vi "Server_Detect.vi"(8 "error in":errorcluster, 11 "Main Update Data":T1) -> (0 "error out":errorcluster)   [LabVIEW 2018, in "Cloud Server.lvlib"]
uses:
  Cloud Server.lvlib
  Data Def/Server_Main Update Data.ctl
  Data Def/Server_Connection Manager Method.ctl
  Com VIs/Data Def/Update Result.ctl
  Data Def/Server_Main Loop Queue Data.ctl
  Data Def/Server_Main Loop State.ctl
  Com VIs/Data Def/Data File Format.ctl
  <vilib>/gmath/NI_Gmath.lvlib
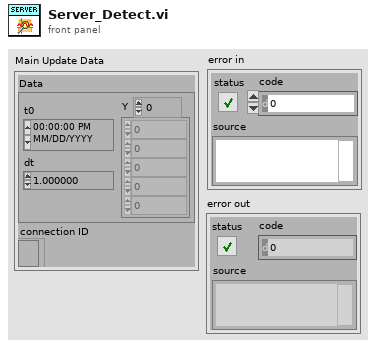
[diagram p1: front panel]
types:
  T1 = typedef "Cloud Server.lvlib/Server_Main Update Data.ctl" = cluster{"Data":waveform(dbl), "connection ID":refnum<k5>}
  T2 = typedef "Cloud Server.lvlib/Server_Connection Manager Method.ctl" = enum16{"Initialize", "Add", "Get", "Set Properties", "Get Properties", "Close", "Release"}
  T3 = typedef "Cloud Server.lvlib/Server_Connection Properties.ctl" = cluster{"User Data":T4, "Data":waveform(dbl)}
  T4 = typedef "User Data.ctl" = cluster{"Name":string, "Email":string, "Phone Number":string, "User Picture":u32[][], "Last Login Time":timestamp}
  T5 = typedef "Update Result.ctl" = enum16{"Normal", "Abnormal", "Can't find training data"}
  T6 = typedef "Data File Format.ctl" = cluster{"Data":waveform(dbl), "Abnormal?":bool, "Measure Time":timestamp, "User Name":string}
  T7 = typedef "Cloud Server.lvlib/Server_Main Loop Queue Data.ctl" = cluster{"Main Loop State":T8, "Data":variant}
  T8 = typedef "Cloud Server.lvlib/Server_Main Loop State.ctl" = enum16{"Detect", "Save", "Training", "Refresh User Name", "Stop"}
  T9 = typedef "Cloud Server.lvlib/Server_Training Data.ctl" = cluster{"Data":waveform(dbl), "Abnormal?":bool}
  T10 = typedef "Cloud Server.lvlib/Server_Main Data.ctl" = cluster{"Main VI Ref.":refnum<vi>, "Listener ID":refnum<k5>, "Meta data":T11[], "Main Queue":T13, "User Picture":T14}
  T11 = typedef "stm_MetaElement.ctl" = cluster{"Name":T12}
  T12 = typedef "stm_MetaDataElement.ctl" = string
  T13 = typedef "Cloud Server.lvlib/Server_Main Queue.ctl" = cluster{"Server Write Queue":refnum<queue>, "Main Loop Queue":refnum<queue>}
  T14 = typedef "IMAQ Image.ctl" = refnum<image>
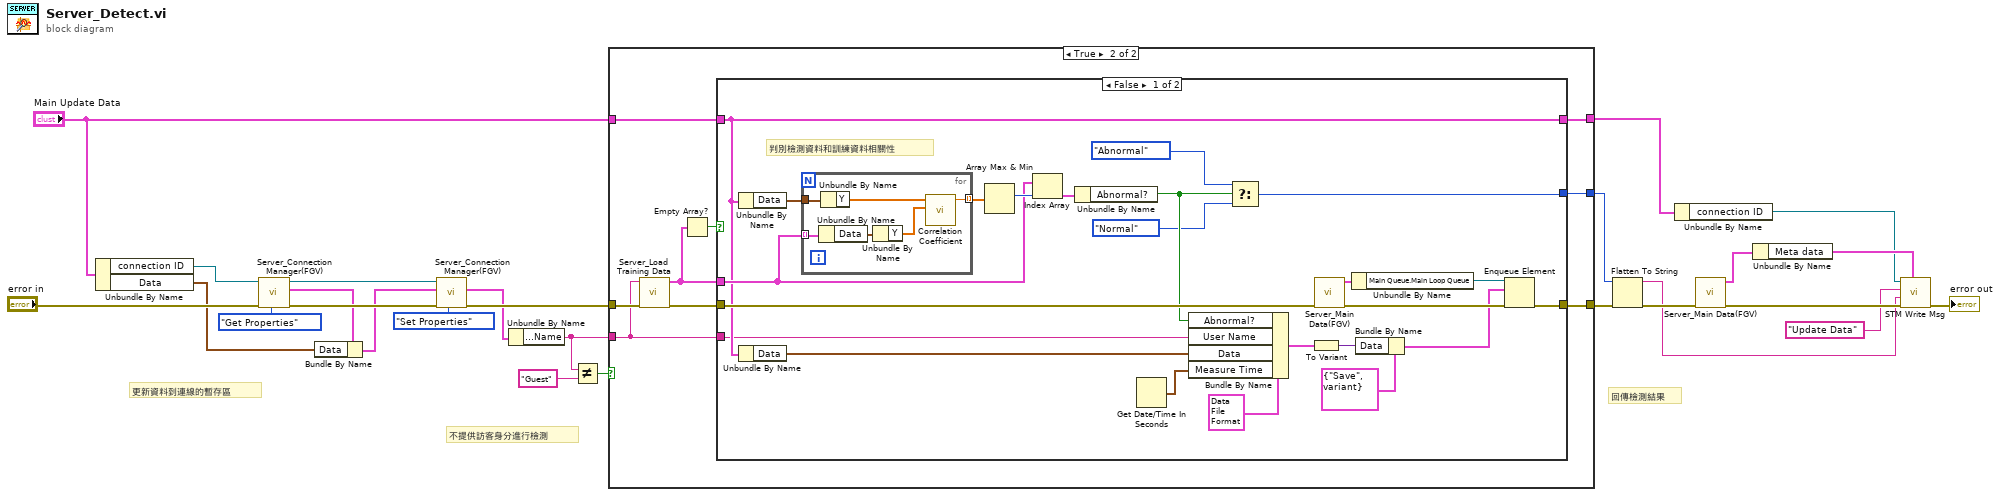
[diagram p0: block diagram]
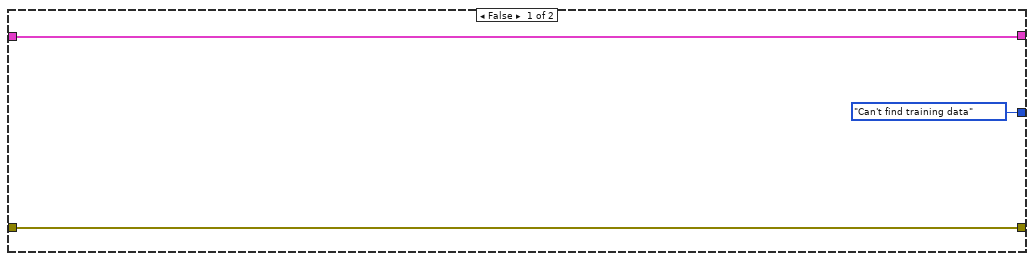
[diagram p2: hidden frame]
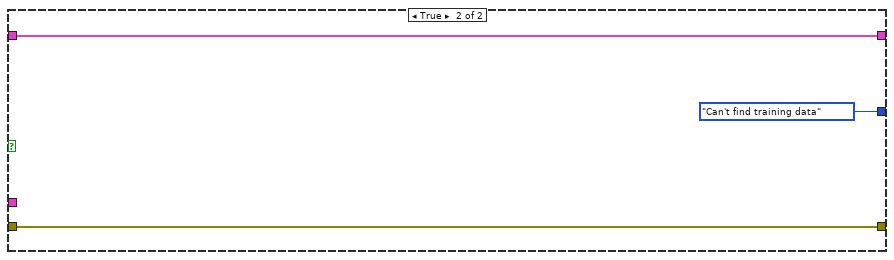
[diagram p3: hidden frame]
diagram:
  # "回傳檢測結果"
  # "不提供訪客身分進行檢測"
  # "更新資料到連線的暫存區"
  n1 = Unbundle By Name("Main Update Data") -> ("connection ID"=w4:refnum<k5>, "Data"=w1:waveform(dbl))
  n2 = call "Server_Connection Manager(FGV).vi"("Connection Manager Method(Get)"=Server_Connection_Manager_Method."Get Properties", "error in"="error in", "Connection In"=w4) -> ("error out"=w10:errorcluster, "Connection Properties Out"=w7:T3, "Connection Out"=w9:refnum<k5>)  [unwired: 4 in, 2 out]
  n3 = Bundle By Name(cluster=w7, "Data"=w1) -> (w6:T3)
  n4 = call "Server_Connection Manager(FGV).vi"("Connection Manager Method(Get)"=Server_Connection_Manager_Method."Set Properties", "error in"=w10, "Connection Properties In"=w6, "Connection In"=w9) -> ("error out"=w5:errorcluster, "Connection Properties Out"=w3:T3)  [unwired: 3 in, 3 out]
  n5 = Unbundle By Name(w3) -> ("User Data.Name"=w24:string)
  n6 = Not Equal?(x=w24, y="Guest" ("x")) -> (x != y?=w25:bool)
  n7 = case shown="True" w25 {
    tunnel: w5 -> [w29 w38]
    tunnel: w24 -> [_ w30]
    tunnel: "Main Update Data" -> [w28 w34]
    tunnel: [Update_Result."Can't find training data" ("Update Result") w33] -> w15
    tunnel: [w29 w32] -> w17
    tunnel: [w28 w31] -> w22
    frame False {
    }
    frame True {
      n8 = call "Server_Load Training Data.vi"("error in"=w38, "Name"=w30) -> ("error out"=w36:errorcluster, "Training Data"=w35:T9[])  [unwired: 8 in]
      n9 = Empty Array?(array=w35) -> (empty?=w37:bool)
      n10 = case shown="False" w37 {
        tunnel: w36 -> [w55 w70]
        tunnel: w35 -> [w58 _]
        tunnel: w34 -> [w49 w69]
        tunnel: [w52 w70] -> w32
        tunnel: [w56 Update_Result."Can't find training data" ("Update Result")] -> w33
        tunnel: [w49 w69] -> w31
        tunnel: w30 -> [w44 _]
        frame False {
          # "判別檢測資料和訓練資料相關性"
          n11 = Unbundle By Name(w49) -> ("Data"=w61:waveform(dbl))
          n12 = Unbundle By Name(w49) -> ("Data"=w43:waveform(dbl))
          n13 = for {
            tunnel: w58 -> [w67] mode=indexing
            tunnel: w61 -> [w66]
            tunnel: [w62] -> w60 mode=indexing
            n14 = Unbundle By Name(w67) -> ("Data"=w65:waveform(dbl))
            n15 = Unbundle By Name(w66) -> ("Y"=w64:dbl[])
            n16 = Unbundle By Name(w65) -> ("Y"=w63:dbl[])
            n17 = call <vilib>:"Correlation Coefficient.vi"("Y"=w63, "X"=w64) -> ("correlation coefficient r"=w62:dbl)  [unwired: 8 in, 1 out]
          }
          n18 = Array Max & Min(array=w60) -> (max index (indices)=w59:i32)  [unwired: 3 out]
          n19 = Index Array(array=w58, index=w59) -> (element=w57:T9)
          n20 = Unbundle By Name(w57) -> ("Abnormal?"=w50:bool)
          n21 = Get Date/Time In Seconds() -> (seconds since 1Jan1904=w42:timestamp)
          n22 = Bundle By Name(cluster=T6 {"Data"={"t0"=timestamp(0 s since 1904-01-01), "dt"=1.0, "Y"=[]}, "Abnormal?"=FALSE, "Measure Time"=timestamp(0 s since 1904-01-01), "User Name"=""} ("Data File Format"), "Abnormal?"=w50, "User Name"=w44, "Data"=w43, "Measure Time"=w42) -> (w48:T6)
          n23 = Select(t=Update_Result."Abnormal" ("Update Result"), s=w50, f=Update_Result."Normal" ("Update Result")) -> (s? t:f=w56:T5)
          n24 = To Variant(anything=w48) -> (Variant=w46:variant)
          n25 = call "Server_Main Data(FGV).vi"("error in"=w55) -> ("error out"=w53:errorcluster, "Main Data Out"=w54:T10)  [unwired: 9 in]
          n26 = Unbundle By Name(w54) -> ("Main Queue.Main Loop Queue"=w51:refnum<queue>)
          n27 = Bundle By Name(cluster=T7 {"Main Loop State"=enum."Save", "Data"=variant} ("element"), "Data"=w46) -> (w45:T7)
          n28 = Enqueue Element(queue=w51, element=w45, error in (no error)=w53) -> (error out=w52:errorcluster)  [unwired: 1 in, 2 out]
        }
        frame True {
        }
      }
    }
  }
  n29 = Flatten To String(anything=w15, error in (no error)=w17) -> (data string=w14:string, error out=w16:errorcluster)  [unwired: 2 in, 1 out]
  n30 = Unbundle By Name(w22) -> ("connection ID"=w18:refnum<k5>)
  n31 = call "Server_Main Data(FGV).vi"("error in"=w16) -> ("error out"=w21:errorcluster, "Main Data Out"=w20:T10)  [unwired: 9 in]
  n32 = Unbundle By Name(w20) -> ("Meta data"=w19:T11[])
  n33 = call "STM Write Msg.vi"("Meta data"=w19, "error in (no error)"=w21, "Data"=w14, "Name"="Update Data", "connection ID"=w18) -> ("error out"=→"error out":errorcluster)  [unwired: 5 in, 1 out]
